vi "Main.vi"(8 "error in":errorcluster, 11 "Worker A in":refnum<class "Worker A.lvclass">) -> (0 "error out":errorcluster, 3 "Worker A out":refnum<class "Worker A.lvclass">)   [LabVIEW 2017, in "Worker A.lvclass"]
doc: "The <b>Queued Message Handler</b> of the Worker that owns this VI."
uses:
  Worker A.lvclass
  Initialization Data.ctl
  Response Cases.ctl
  Worker A.lvclass/Worker A.ctl
  rql_Generate Error.ctl
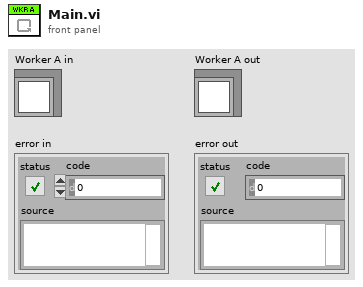
[diagram p1: front panel]
types:
  T1 = typedef "Worker A.lvclass/Initialization Data.ctl" = cluster{"Response Cases":T2}
  T2 = typedef "Worker A.lvclass/Response Cases.ctl" = cluster{"Placeholder - Can be deleted":string}
  T3 = typedef "Worker A.lvclass/rql_Generate Error.ctl" = cluster{"String":string}
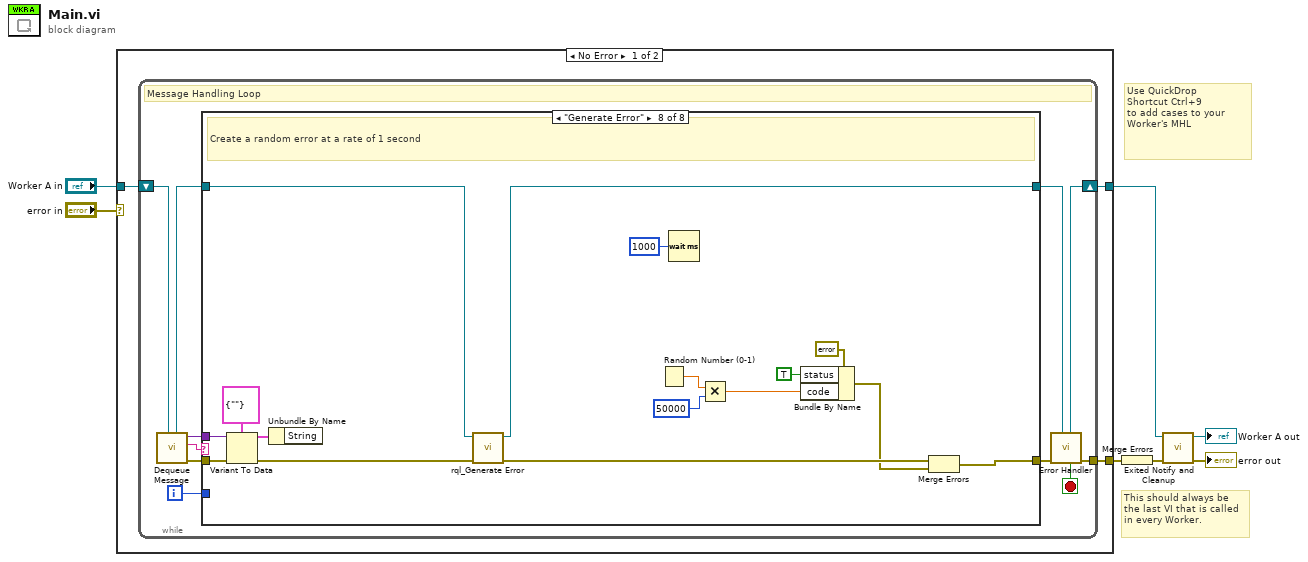
[diagram p0: block diagram]
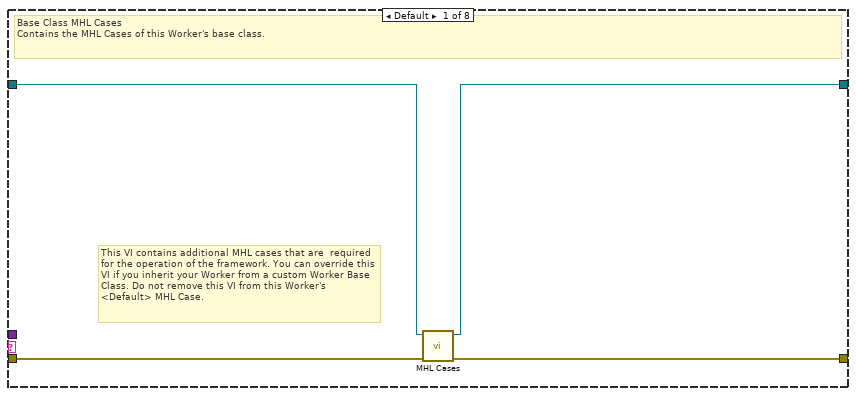
[diagram p2: hidden frame]
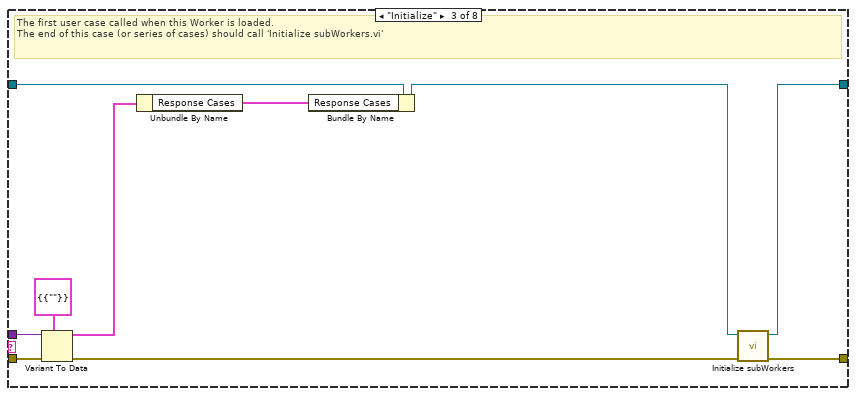
[diagram p4: hidden frame]
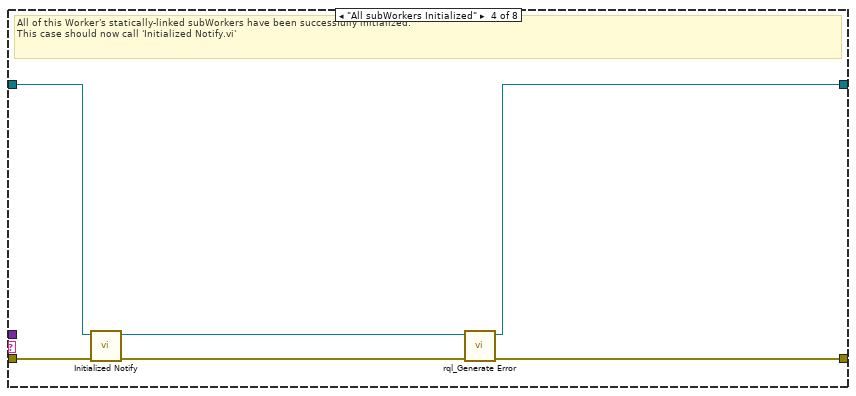
[diagram p5: hidden frame]
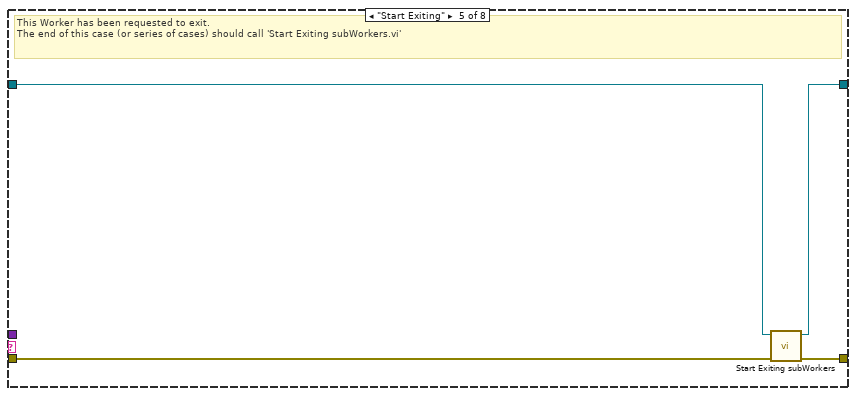
[diagram p6: hidden frame]
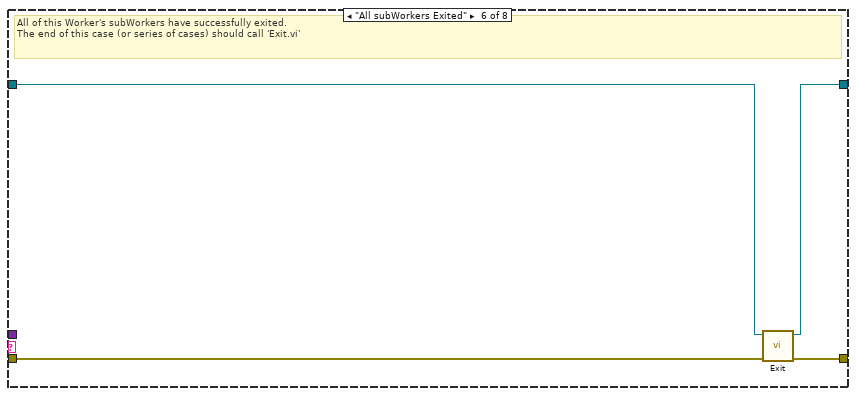
[diagram p7: hidden frame]
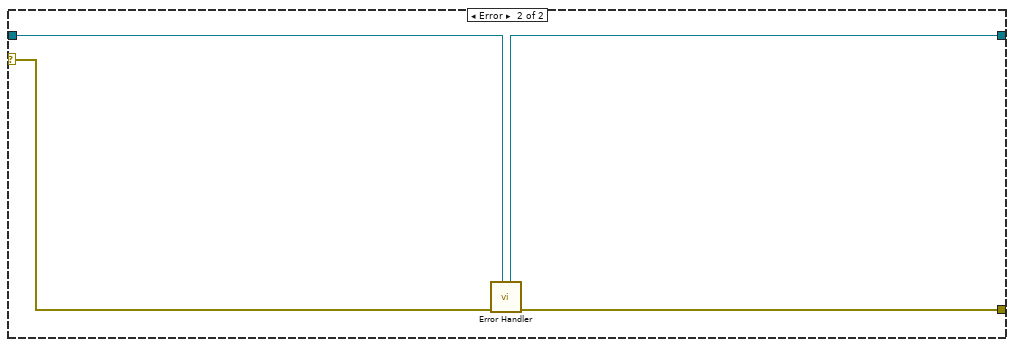
[diagram p9: hidden frame]
diagram:
  # "Use QuickDrop\nShortcut Ctrl+9\nto add cases to your\nWorker's MHL"
  # "This should always be the last VI that is called in every Worker."
  n1 = case shown="No Error" "error in" {
    tunnel: "Worker A in" -> [w10 w71]
    tunnel: [w8 w72] -> w5
    tunnel: [w9 w70] -> w6
    selector: "error in" -> [_ w73]
    frame No Error {
      n2 = while {
        shift-right: [w19] -> w9
        shift-left: w10 -> [w21]
        tunnel: [w20] -> w8
        i -> [w12]
        stop <- w13 stop-if-true
        # "Message Handling Loop"
        n3 = call-dynamic "Dequeue Message.vi"("Worker"=w21) -> ("error out"=w18:errorcluster, "Case out"=w14:string, "Data out"=w11:variant, "Worker out"=w16:refnum<class "Worker A.lvclass">)  [unwired: 6 in, 1 out]
        n4 = case "Worker MHL Case Structure (DO NOT CHANGE LABEL NAME)" shown="\"Generate Error\"" w14 {
          tunnel: w18 -> [w25 w26 w35 w42 w44 w51 w53 w69]
          tunnel: [w24 w26 w37 w40 w47 w50 w53 w56] -> w17
          tunnel: w16 -> [w23 w27 w34 w43 w45 w49 w52 w63]
          tunnel: [w22 w27 w36 w38 w46 w48 w52 w62] -> w15
          tunnel: w12 -> [_ _ _ _ _ _ _ _]
          tunnel: w11 -> [_ _ w32 _ _ _ _ w66]
          frame Default {
            # "This VI contains additional MHL cases that are  required for the operation of the framework. You can override this VI if you inherit your Worker from a custom Worker Base Class. Do not remove this VI from this Worker's <Default> MHL Case."
            # "Base Class MHL Cases\nContains the MHL Cases of this Worker's base class."
            n5 = call-dynamic "MHL Cases.vi"("error in"=w25, "Worker in"=w23) -> ("error out"=w24:errorcluster, "Worker out"=w22:refnum<class "Worker A.lvclass">)  [unwired: 8 in]
          }
          frame "------------ FRAMEWORK CASES -----------" {
            # "Start of Workers Framework Cases"
          }
          frame "Initialize" {
            # "The first user case called when this Worker is loaded.\nThe end of this case (or series of cases) should call 'Initialize subWorkers.vi'"
            n6 = Variant To Data(error in=w35, type=T1 {"Response Cases"={"Placeholder - Can be deleted"=""}} ("Initialization Data"), Variant=w32) -> (data=w30:T1, error out=w33:errorcluster)
            n7 = Unbundle By Name(w30) -> ("Response Cases"=w29:T2)
            n8 = Bundle By Name(cluster=w34, "Response Cases"=w29) -> (w31:refnum<class "Worker A.lvclass">)
            n9 = call-dynamic "Initialize subWorkers.vi"("error in"=w33, "Worker"=w31) -> ("error out"=w37:errorcluster, "dup Worker out"=w36:refnum<class "Worker A.lvclass">)  [unwired: 8 in]
          }
          frame "All subWorkers Initialized" {
            # "All of this Worker's statically-linked subWorkers have been successfully initialized.\nThis case should now call 'Initialized Notify.vi'"
            n10 = call-dynamic "Initialized Notify.vi"("error in"=w42, "Worker"=w43) -> ("error out"=w41:errorcluster, "dup Worker out"=w39:refnum<class "Worker A.lvclass">)  [unwired: 8 in]
            n11 = call "rql_Generate Error.vi"("error in"=w41, "Worker A in"=w39) -> ("error out"=w40:errorcluster, "dup Worker A out"=w38:refnum<class "Worker A.lvclass">)  [unwired: 8 in]
          }
          frame "Start Exiting" {
            # "This Worker has been requested to exit. \nThe end of this case (or series of cases) should call 'Start Exiting subWorkers.vi'"
            n12 = call-dynamic "Start Exiting subWorkers.vi"("error_in"=w44, "Worker"=w45) -> ("error out"=w47:errorcluster, "dup Worker out"=w46:refnum<class "Worker A.lvclass">)  [unwired: 8 in]
          }
          frame "All subWorkers Exited" {
            # "All of this Worker's subWorkers have successfully exited. \nThe end of this case (or series of cases) should call 'Exit.vi'"
            n13 = call-dynamic "Exit.vi"("error_in"=w51, "Worker"=w49) -> ("error out"=w50:errorcluster, "dup Worker out"=w48:refnum<class "Worker A.lvclass">)  [unwired: 8 in]
          }
          frame "------------- LOCAL API CASES -------------" {
            # "Start of Workers Local API Cases"
          }
          frame "Generate Error" {
            # "Create a random error at a rate of 1 second"
            n14 = Variant To Data(error in=w69, type=T3 {"String"=""} ("Data"), Variant=w66) -> (data=w65:T3, error out=w68:errorcluster)
            n15 = Unbundle By Name(w65) -> ()  [unwired: 1 out]
            n16 = call "rql_Generate Error.vi"("error in"=w68, "Worker A in"=w63) -> ("error out"=w64:errorcluster, "dup Worker A out"=w62:refnum<class "Worker A.lvclass">)  [unwired: 8 in]
            n17 = Random Number (0-1)() -> (number: 0 to 1=w59:dbl)
            n18 = Wait (ms)(milliseconds to wait=u32 1000) -> ()  [unwired: 1 out]
            n19 = Multiply(x=w59, y=50000) -> (x*y=w57:dbl)
            n20 = Bundle By Name(cluster=errorcluster {"status"=TRUE, "code"=0, "source"=""} ("error constant"), "status"=TRUE, "code"=w57) -> (w54:errorcluster)
            n21 = Merge Errors(w64, w54) -> (w56:errorcluster)
          }
        }
        n22 = call-dynamic "Error Handler.vi"("Worker A"=w15, "error_in"=w17) -> ("error out"=w20:errorcluster, "Stop Loop"=w13:bool, "Worker A out"=w19:refnum<class "Worker A.lvclass">)  [unwired: 7 in]
      }
    }
    frame Error {
      n23 = call-dynamic "Error Handler.vi"("Worker A"=w71, "error_in"=w73) -> ("error out"=w72:errorcluster, "Worker A out"=w70:refnum<class "Worker A.lvclass">)  [unwired: 7 in, 1 out]
    }
  }
  n24 = Merge Errors(w5) -> (w7:errorcluster)
  n25 = call-dynamic "Exited Notify and Cleanup.vi"("error_in"=w7, "Worker"=w6) -> ("error out"=→"error out":errorcluster, "dup Worker out"=→"Worker A out":refnum<class "Worker A.lvclass">)  [unwired: 8 in]
